vi "FullContrast.vi"(0 "LightField Automation":refnum<class "LightField Automation.lvclass">, 1 "PZC200 Instrument Channel":string="GPIB/0:4,0", 2 "ExcWL_nm":dbl, 3 "PZC Error":errorcluster, 4 "Acq Time (ms) 2":dbl=500.0 caption="Acq Time :" min=0.0 max=360000.0 step=50.0, 5 "Acq Mode":T1=enum."Spectrum" caption="Mode :", 6 "CCD ROI":T2(ring), 7 "LightField Automation error":errorcluster, 8 "Shutter Device Reference":refnum<vi>, 9 "PZC Position Readout (usteps) 2":refnum<vi>, 10 "LinTFine Start":dbl, 11 "LinTFine End":dbl, 12 "Shutter Controls":refnum<vi>, 13 "Scan Spectrum Progess Bar 2":refnum<vi>, 14 "Stop Contrast 2":refnum<vi>, 15 "Pause Contrast 2":refnum<vi>, 16 "Contrast 1D Spectrum 2":refnum<vi>, 17 "LinTFine Step":dbl, 18 "Accumulations":dbl=1.0, 19 "Contrast Oscillations 2":refnum<vi>, 22 "Photodiode handle out":refnum<visa-resource-name> caption="instrument handle out", 23 "Photodiode error out":errorcluster caption="error out" {"code" format="%.0x"}) -> (20 "LightField Automation out":refnum<class "LightField Automation.lvclass">, 21 "PZC200 Instrument Channel 2":string, 24 "PZC Error 2":errorcluster, 25 "PZAPos & InstPow":dbl[][](array[numeric]), 26 "Spectra vs PZA":i32[][](array[numeric]), 27 "LightField Automation error  out":errorcluster)   [LabVIEW 2019]
uses:
  D:/Users/manip-thz/Documents/Controle_Manip_2020/Thorlabs.MotionControl.KCube.SolenoidCLI.dll
  Thorlabs.MotionControl.KCube.SolenoidCLI.dll
  Light Field/lightfield-automation-labview/LightField Automation.lvclass
  TypeDefs/AcqMode.ctl
panel:
  out "InstPow":dbl[](array[numeric])
  out "ExcPow_uW":dbl
  out "WavelengthCalibration":dbl[](array[numeric])
  out "x+y":dbl
  out "PZA Positions":i32[](array[numeric])
  out "Contrast values":i32[](array[numeric])
  out "Contrast 1D Spectrum":cluster{dbl[], dbl[]}(graph) caption="64.0°"
  out "Contrast Oscillations":cluster{dbl[], dbl[]}(graph)
  in  "Pause Contrast":bool
  in  "Stop Contrast":bool
  out "PZC Position Readout (usteps)":dbl caption="Readout (usteps)" min=-8.0 max=392.0
  out "Scan Spectrum Progess Bar":u8(slide) scale=0.0..100.0
  out "KCube Shutter Device Reference":refnum<k24>
  out "Shutter Ctrls":u16(ring)
  # "ms"
types:
  T1 = typedef "AcqMode.ctl" = enum16{"Image", "Spectrum", "APD 1", "APD 2", "APD 1+2"}
  T2 = enum16{"Custom ROI", "Full sensor", "Binned full sensor"}
  T3 = enum16{"Contrast", "Spectre", "Polarisation", "XY Intensity Map"}
  T4 = enum16{"Image", "Spectrum", "APD 1", "APD 2", "APD 1+2"}
  T5 = cluster{"Image":dbl[][][], "Frame Size":cluster{"F":i32, "Y":i32, "X":i32}}[]
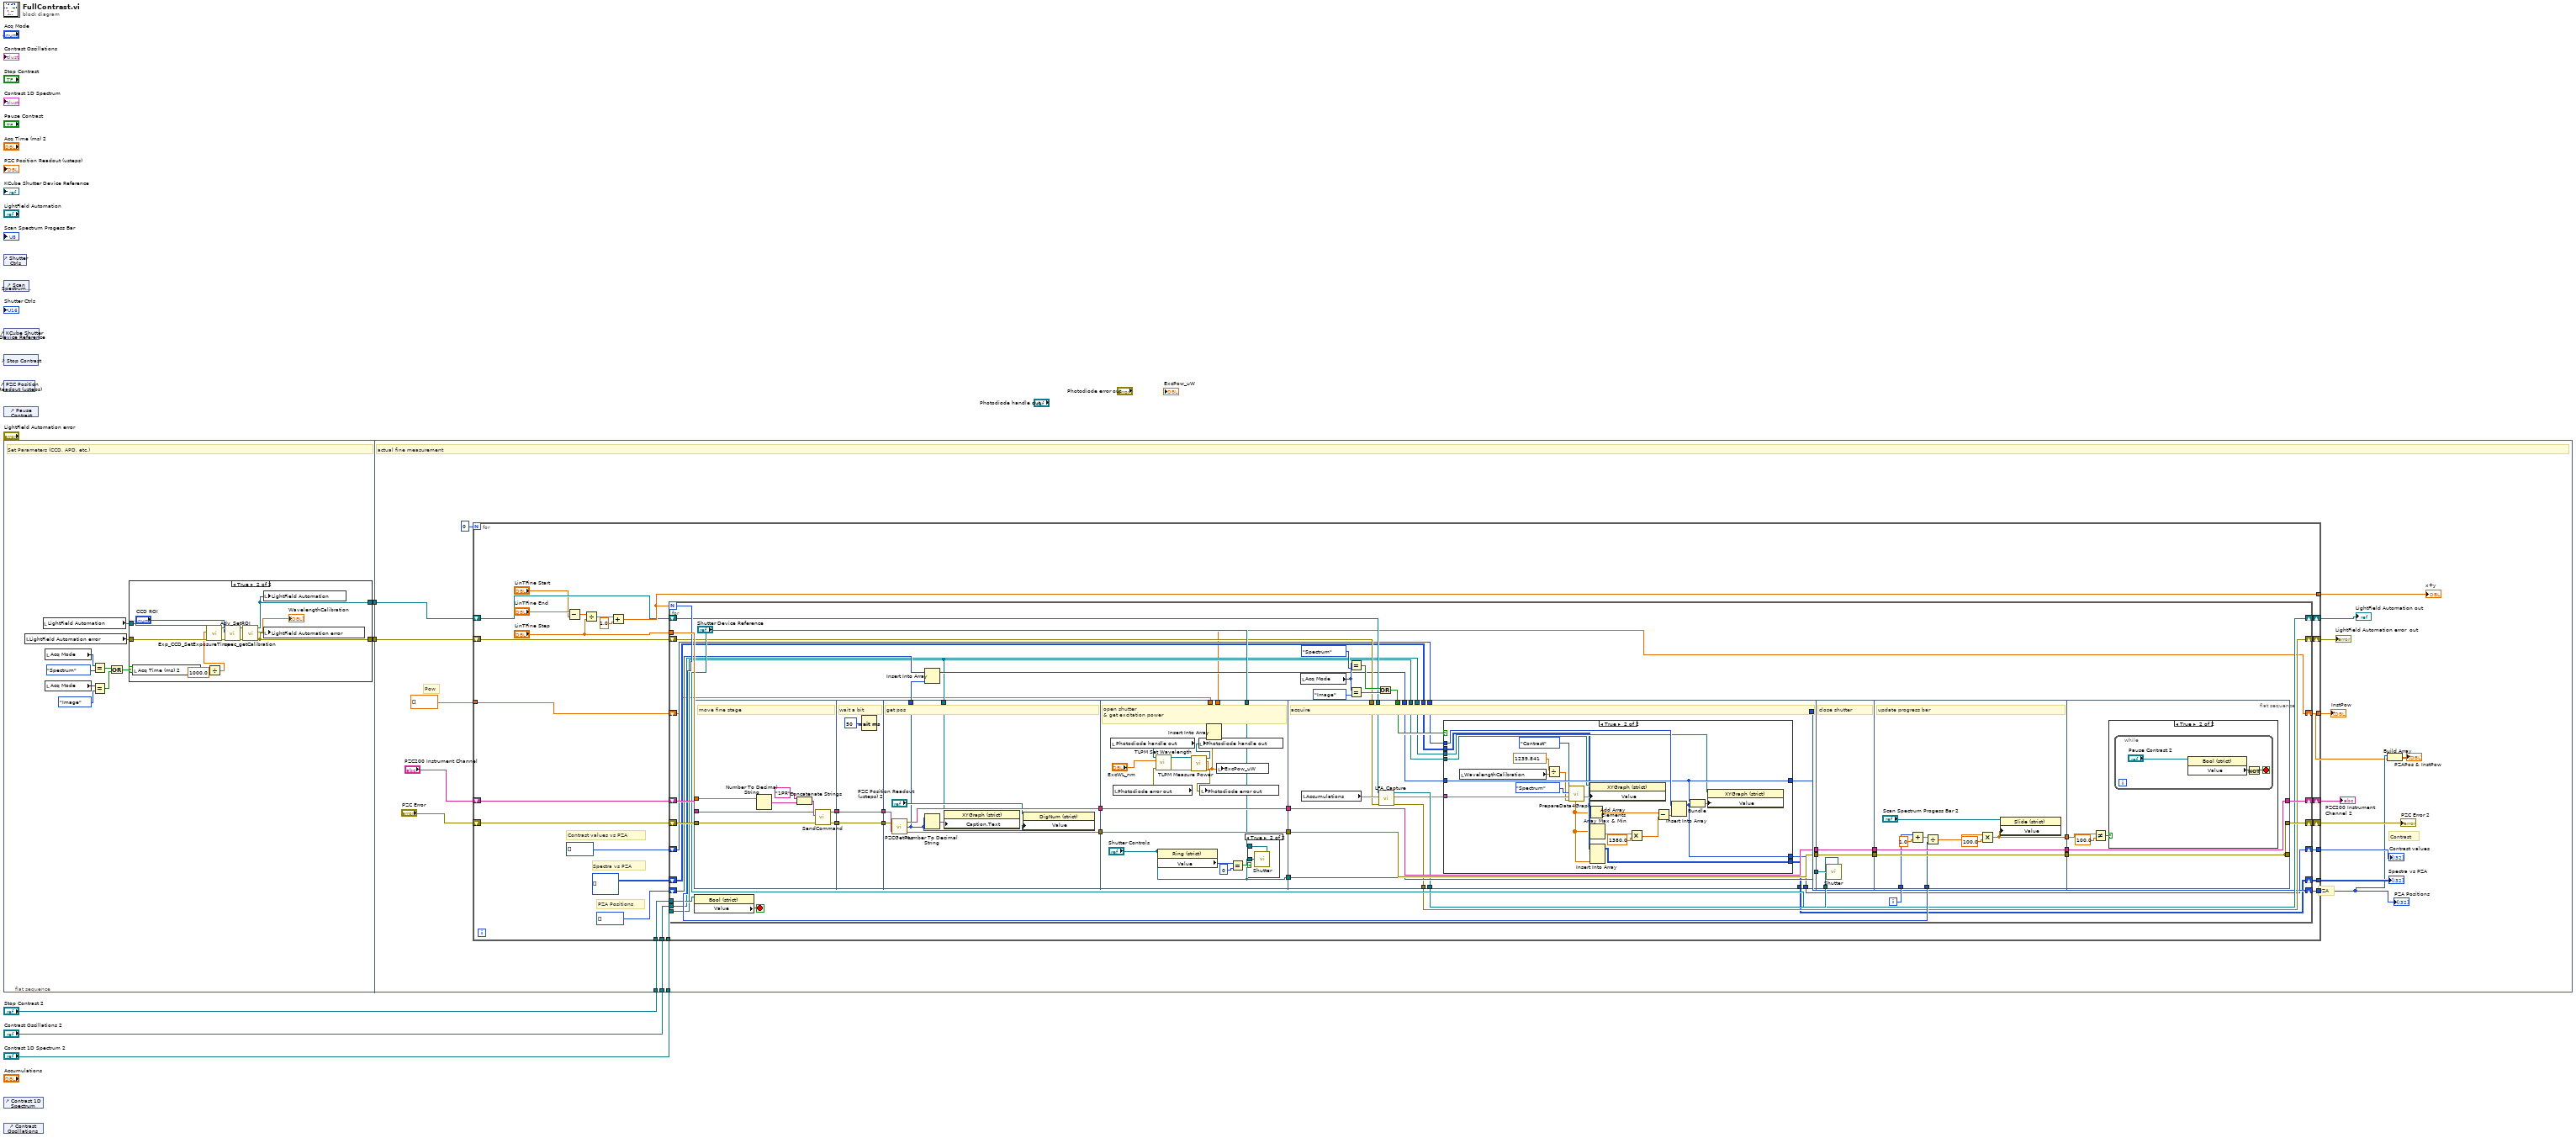
[diagram p0: block diagram]
diagram:
  n1 = control-ref of="Shutter Ctrls"() -> ()  [unwired: 1 out]
  n2 = control-ref of="Scan Spectrum Progess Bar"() -> ()  [unwired: 1 out]
  n3 = control-ref of="KCube Shutter Device Reference"() -> ()  [unwired: 1 out]
  n4 = control-ref of="Stop Contrast"() -> ()  [unwired: 1 out]
  n5 = control-ref of="PZC Position Readout (usteps)"() -> ()  [unwired: 1 out]
  n6 = control-ref of="Pause Contrast"() -> ()  [unwired: 1 out]
  n7 = flat-sequence {
    tunnel: [w9] -> w5
    tunnel: [w8] -> w4
    tunnel: w5 -> [w45]
    tunnel: w4 -> [w44]
    tunnel: "Stop Contrast 2" -> [w40]
    tunnel: "Contrast 1D Spectrum 2" -> [w39]
    tunnel: "Contrast Oscillations 2" -> [w38]
    frame #0 {
      # "Set Parameters (CCD, APD, etc.)"
      n8 = local read "LightField Automation error"() -> (w7:errorcluster)
      n9 = local read "LightField Automation"() -> (w6:refnum<class "LightField Automation.lvclass">)
      n10 = local read "Acq Mode"() -> (w16:T1)
      n11 = local read "Acq Mode"() -> (w12:T1)
      n12 = Equal?(x=w16, y=AcqMode."Spectrum" ("Acq Mode")) -> (x = y?=w14:bool)
      n13 = Equal?(x=w12, y=AcqMode."Image" ("Acq Mode")) -> (x = y?=w11:bool)
      n14 = Or(x=w14, y=w11) -> (x .or. y?=w10:bool)
      n15 = case shown="True" w10 {
        tunnel: [w18 w24] -> w9
        tunnel: [w17 w23] -> w8
        tunnel: w7 -> [w17 w28]
        tunnel: w6 -> [w18 w27]
        frame False {
        }
        frame True {
          n16 = local read "Acq Time (ms) 2"() -> (w21:dbl)
          n17 = Divide(x=w21, y=1000.0) -> (x/y=w19:dbl)
          n18 = call "Exp_CCD_SetExposureTime.vi"("error in (no error)"=w28, "Exposure Time (s)"=w19, "LightField Automation in"=w27) -> ("error out"=w30:errorcluster, "LightField Automation out"=w31:refnum<class "LightField Automation.lvclass">)  [unwired: 7 in]
          n19 = call "Adv_SetROI.vi"("error in (no error)"=w30, "ROI"="CCD ROI", "LightField Automation in"=w31) -> ("error out"=w25:errorcluster, "LightField Automation out"=w26:refnum<class "LightField Automation.lvclass">)  [unwired: 7 in]
          n20 = call "spec_getCalibration.vi"("error in (no error)"=w25, "LightField Automation in"=w26) -> ("error out"=w23:errorcluster, "ColumnCalibration"=→"WavelengthCalibration":dbl[], "LightField Automation out"=w24:refnum<class "LightField Automation.lvclass">)  [unwired: 7 in]
          n21 = local write "LightField Automation"(w24) -> ()
          n22 = local write "LightField Automation error"(w23) -> ()
        }
      }
    }
    frame #1 {
      # "Pow"
      # "Contrast"
      # "PZA"
      # "actual fine measurement"
      n23 = for {
        N: 0 -> [_]
        tunnel: [w76] -> w50
        tunnel: [w64] -> w41
        tunnel: w40 -> [w63]
        tunnel: w39 -> [w62]
        tunnel: w38 -> [w61]
        tunnel: [w59] -> w37
        tunnel: dbl[] [] -> [w58]
        tunnel: [w57] -> w35
        tunnel: [w56] -> w34
        shift-right: [w71] -> w46
        shift-left: "PZC Error" -> [w74]
        shift-right: [w72] -> w47
        shift-left: "PZC200 Instrument Channel" -> [w73]
        shift-right: [w68] -> w43
        shift-left: w45 -> [w70]
        shift-right: [w67] -> w42
        shift-left: w44 -> [w69]
        # "Spectra vs PZA"
        # "Contrast values vs PZA"
        # "PZA Positions"
        n24 = Subtract(x="LinTFine End", y="LinTFine Start") -> (x-y=w53:dbl)
        n25 = Divide(x=w53, y="LinTFine Step") -> (x/y=w52:dbl)
        n26 = Add(x=w52, y=1.0) -> (x+y=w76:dbl)
        n27 = for {
          N: w76 -> [w109]
          tunnel: "LinTFine Step" -> [w125]
          shift-right: [w104] -> w72
          shift-left: w73 -> [w123]
          shift-right: [w103] -> w71
          shift-left: w74 -> [w124]
          shift-right: [w92] -> w68
          shift-left: w70 -> [w94]
          shift-right: [w91] -> w67
          shift-left: w69 -> [w93]
          shift-right: [w81] -> w57
          shift-left: i32[] [] -> [w89]
          shift-right: [w80] -> w64
          shift-left: i32[] [] -> [w86]
          tunnel: w63 -> [w88]
          tunnel: w62 -> [w84]
          tunnel: w61 -> [w83]
          shift-right: [w79] -> w59
          shift-left: i32[][] [] -> [w82]
          shift-right: [w77] -> w56
          shift-left: w58 -> [w78]
          i -> [w110]
          stop <- w105 stop-if-true
          n28 = flat-sequence {
            tunnel: w125 -> [w133]
            tunnel: [w129] -> w122
            tunnel: [w128] -> w120
            tunnel: w124 -> [w127]
            tunnel: w123 -> [w126]
            tunnel: w122 -> [w136]
            tunnel: [w136] -> w121
            tunnel: w120 -> [w135]
            tunnel: [w135] -> w119
            tunnel: w121 -> [w144]
            tunnel: w119 -> [w143]
            tunnel: [w142] -> w118
            tunnel: [w141] -> w117
            tunnel: [w137] -> w90
            tunnel: w84 -> [w139]
            tunnel: w118 -> [w161]
            tunnel: w117 -> [w160]
            tunnel: "Shutter Device Reference" -> [w156]
            tunnel: [w161] -> w116
            tunnel: [w160] -> w115
            tunnel: ["Shutter Controls"] -> w101
            tunnel: w78 -> [w147]
            tunnel: [w145] -> w77
            tunnel: w116 -> [w181]
            tunnel: w115 -> [w180]
            tunnel: [w181] -> w114
            tunnel: [w180] -> w113
            tunnel: [w178] -> w102
            tunnel: w101 -> [w178]
            tunnel: w94 -> [w177]
            tunnel: w93 -> [w176]
            tunnel: [w175] -> w92
            tunnel: [w174] -> w91
            tunnel: w87 -> [w173]
            tunnel: w86 -> [w171]
            tunnel: w85 -> [w170]
            tunnel: w84 -> [w169]
            tunnel: w83 -> [w168]
            tunnel: w82 -> [w167]
            tunnel: [w166] -> w81
            tunnel: [w165] -> w80
            tunnel: [w164] -> w79
            tunnel: w114 -> [w209]
            tunnel: w113 -> [w208]
            tunnel: [w209] -> w112
            tunnel: [w208] -> w111
            tunnel: w102 -> [w207]
            tunnel: "Shutter Device Reference" -> [w206]
            tunnel: w112 -> [w219]
            tunnel: w111 -> [w218]
            tunnel: w110 -> [w212]
            tunnel: w109 -> [w211]
            tunnel: [w219] -> w108
            tunnel: [w218] -> w107
            tunnel: [w210] -> w106
            tunnel: [w220] -> _
            tunnel: [w224] -> w104
            tunnel: w108 -> [w224]
            tunnel: w107 -> [w220]
            tunnel: w106 -> [w222]
            tunnel: [w220] -> w103
            frame #0 {
              # "move fine stage"
              n29 = Number To Decimal String(number=w133) -> (decimal integer string=w131:string)  [unwired: 1 in]
              n30 = Concatenate Strings("1PR", w131) -> (w130:string)
              n31 = call "SendCommand.vi"("error in"=w127, "Command"=w130, "Instrument Channel"=w126) -> ("error out"=w128:errorcluster, "Instrument Channel out"=w129:string)  [unwired: 7 in]
            }
            frame #1 {
              # "wait a bit"
              n32 = Wait (ms)(milliseconds to wait=u32 50) -> ()  [unwired: 1 out]
            }
            frame #2 {
              # "get pos"
              n33 = call "PZCGetPos.vi"("error in"=w143, "Instrument Channel"=w144) -> ("Instrument Channel Out"=w142:string, "Position"=w137:i32, "error out"=w141:errorcluster)
              n34 = Number To Decimal String(number=w137) -> (decimal integer string=w138:string)  [unwired: 1 in]
              n35 = property class="XYGraph (strict)"(reference=w139, "Caption.Text"=w138) -> ()  [unwired: 1 in, 2 out]
              n36 = property class="DigNum (strict)"(reference="PZC Position Readout (usteps) 2", "Value"=w137) -> ()  [unwired: 1 in, 2 out]
            }
            frame #3 {
              # "open shutter\n& get excitation power"
              n37 = local read "Photodiode handle out"() -> (w151:refnum<visa-resource-name>)
              n38 = local read "Photodiode error out"() -> (w152:errorcluster)
              n39 = call <instrlib>:"TLPM Set Wavelength.vi"("error in (no error)"=w152, "Wavelength (0.0)"="ExcWL_nm", "instrument handle"=w151) -> ("error out"=w153:errorcluster, "instrument handle out"=w154:refnum<visa-resource-name>)  [unwired: 7 in]
              n40 = property class="Ring (strict)"(reference="Shutter Controls") -> ("Value"=w157:u16)  [unwired: 1 in, 2 out]
              n41 = call <instrlib>:"TLPM Measure Power.vi"("error in (no error)"=w153, "instrument handle"=w154) -> ("error out"=w148:errorcluster, "Power"=w146:dbl, "instrument handle out"=w149:refnum<visa-resource-name>)  [unwired: 7 in]
              n42 = local write "Photodiode handle out"(w149) -> ()
              n43 = local write "Photodiode error out"(w148) -> ()
              n44 = Insert Into Array(array=w147, new element=w146) -> (w145:dbl[])  [unwired: 1 in]
              n45 = local write "ExcPow_uW"(w146) -> ()
              n46 = Equal?(x=w157, y=u16 0) -> (x = y?=w158:bool)
              n47 = case shown="True" w158 {
                tunnel: "Shutter Controls" -> [_ w163]
                tunnel: w156 -> [_ w162]
                frame False {
                }
                frame True {
                  n48 = call "Shutter.vi"("KCube Shutter Device Reference 2"=w162, "Shutter Ctrls 2"=w163) -> ()
                }
              }
            }
            frame #4 {
              # "acquire"
              n49 = local read "Accumulations"() -> (w179:dbl)
              n50 = call "LFA_Capture.vi"("error in (no error)"=w176, "Frames"=w179, "LightField Automation in"=w177) -> ("error out"=w174:errorcluster, "Data"=w172:T5, "LightField Automation out"=w175:refnum<class "LightField Automation.lvclass">)  [unwired: 6 in]
              n51 = case shown="True" w173 {
                tunnel: w172 -> [_ w205]
                tunnel: w171 -> [w183 w204]
                tunnel: w170 -> [w184 w202]
                tunnel: [w184 w202] -> w166
                tunnel: [w183 w201] -> w165
                tunnel: w169 -> [_ w200]
                tunnel: w168 -> [_ w199]
                tunnel: w167 -> [w182 w195]
                tunnel: [w182 w194] -> w164
                frame False {
                }
                frame True {
                  n52 = local read "WavelengthCalibration"() -> (w187:dbl[])
                  n53 = Divide(x=1239.841, y=w187) -> (x/y=w185:dbl[])
                  n54 = call "PrepareData4Graph.vi"("Wavelength nm"=w185, "DataLF"=w205, "AcqMode"=T4."Spectrum", "Data type"=T3."Contrast") -> ("Spectrum"=w196:cluster{"Array 2":dbl[], "Array":dbl[]}, "PLInt out"=w190:dbl[])  [unwired: 2 in, 2 out]
                  n55 = Add Array Elements(numeric array=w190) -> (sum=w193:dbl)
                  n56 = property class="XYGraph (strict)"(reference=w200, "Value"=w196) -> ()  [unwired: 1 in, 2 out]
                  n57 = Array Max & Min(array=w190) -> (min value=w189:dbl)  [unwired: 3 out]
                  n58 = Insert Into Array(array=w195, new element=w190) -> (w194:i32[][])  [unwired: 2 in]
                  n59 = Multiply(x=w189, y=1380.0) -> (x*y=w188:dbl)
                  n60 = Subtract(x=w193, y=w188) -> (x-y=w192:dbl)
                  n61 = Insert Into Array(array=w204, new element=w192) -> (w201:i32[])  [unwired: 1 in]
                  n62 = Bundle(w202, w201) -> (w203:cluster{i32[], i32[]})  [unwired: 1 in]
                  n63 = property class="XYGraph (strict)"(reference=w199, "Value"=w203) -> ()  [unwired: 1 in, 2 out]
                }
              }
            }
            frame #5 {
              # "close shutter"
              n64 = call "Shutter.vi"("KCube Shutter Device Reference 2"=w206, "Shutter Ctrls 2"=w207) -> ()
            }
            frame #6 {
              # "update progress bar"
              n65 = Add(x=w212, y=1.0) -> (x+y=w216:dbl)
              n66 = Divide(x=w216, y=w211) -> (x/y=w215:dbl)
              n67 = Multiply(x=w215, y=100.0) -> (x*y=w210:dbl)
              n68 = property class="Slide (strict)"(reference="Scan Spectrum Progess Bar 2", "Value"=w210) -> ()  [unwired: 1 in, 2 out]
            }
            frame #7 {
              n69 = Not Equal?(x=w222, y=100.0) -> (x != y?=w221:bool)
              n70 = case shown="True" w221 {
                frame False {
                }
                frame True {
                  n71 = while {
                    stop <- w226 stop-if-true
                    n72 = property class="Bool (strict)"(reference="Pause Contrast 2") -> ("Value"=w227:bool)  [unwired: 1 in, 2 out]
                    n73 = Not(x=w227) -> (.not. x?=w226:bool)
                  }
                }
              }
            }
          }
          n74 = property class="Bool (strict)"(reference=w88) -> ("Value"=w105:bool)  [unwired: 1 in, 2 out]
          n75 = Insert Into Array(array=w89, new element=w90) -> (w85:i32[])  [unwired: 1 in]
          n76 = local read "Acq Mode"() -> (w99:T1)
          n77 = Equal?(x=w99, y=AcqMode."Spectrum" ("Acq Mode")) -> (x = y?=w95:bool)
          n78 = Equal?(x=w99, y=AcqMode."Image" ("Acq Mode")) -> (x = y?=w96:bool)
          n79 = Or(x=w95, y=w96) -> (x .or. y?=w87:bool)
        }
      }
      "LightField Automation out" <- w43
      "LightField Automation error  out" <- w42
      "Contrast values" <- w41
      "PZA Positions" <- w35
      "PZC Error 2" <- w46
      "PZC200 Instrument Channel 2" <- w47
      "x+y" <- w50
      "Spectra vs PZA" <- w37
      "InstPow" <- w34
      n80 = Build Array(w35, w34) -> (→"PZAPos & InstPow":dbl[][])
    }
  }
  n81 = control-ref of="Contrast 1D Spectrum"() -> ()  [unwired: 1 out]
  n82 = control-ref of="Contrast Oscillations"() -> ()  [unwired: 1 out]
